vi "LoggingHeaders.vi"(7 "Match Number":u32, 8 "error in":errorcluster, 9 "Battery Number":string, 10 "Date and Time":string, 11 "refnum in":refnum<file>) -> (0 "error out":errorcluster, 3 "refnum out":refnum<file>)   [LabVIEW 2017]
uses:
  <vilib>/Rock Robotics/Network Tables/NT Read Number.vi
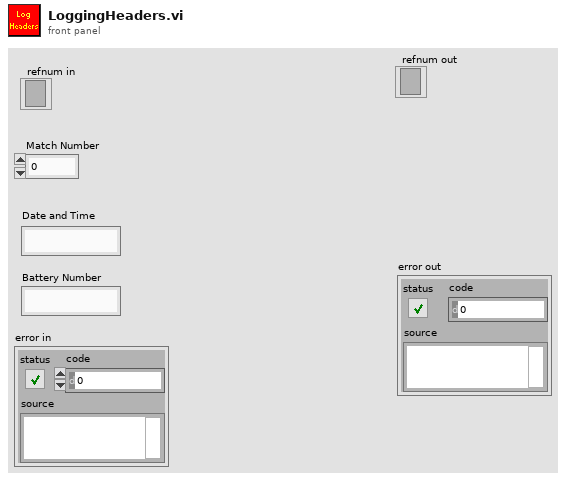
[diagram p1: front panel]
types:
  T1 = typedef "NetComm_MatchType.ctl" = enum32{"None", "Practice", "Qualification", "Elimination"}
  T2 = typedef "WPI_DriverStationPositionInfo.ctl" = enum16{"1", "2", "3"}
  T3 = typedef "WPI_DriverStationAllianceInfo.ctl" = enum16{"Red", "Blue", "Invalid"}
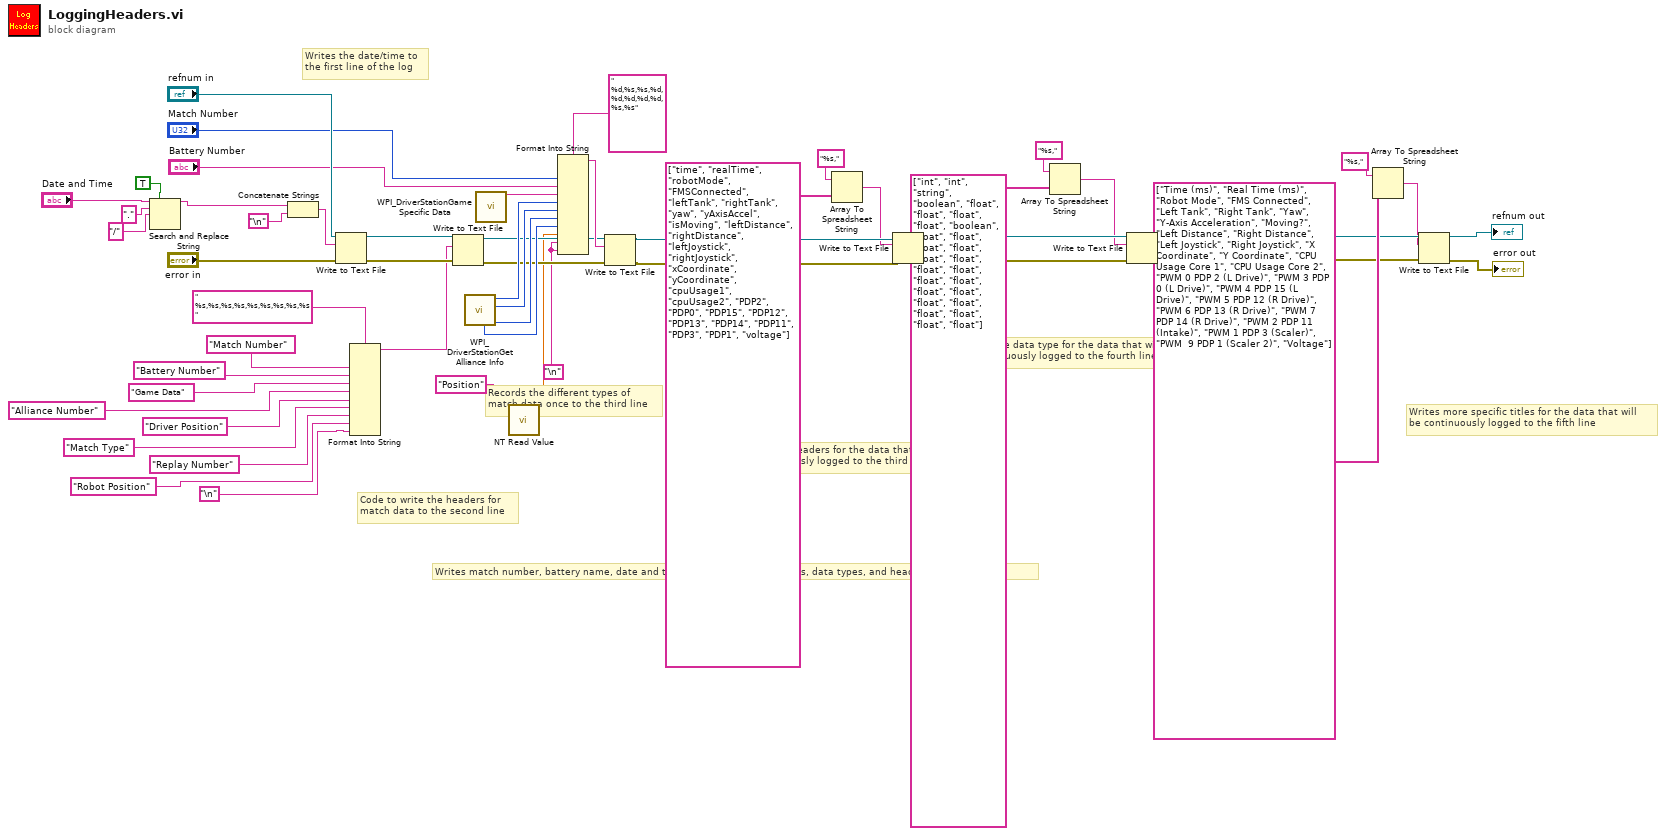
[diagram p0: block diagram]
diagram:
  w1 = "\n"
  # "Writes more specific titles for the data that will \nbe continuously logged to the fifth line"
  # "Writes the data type for the data that will \nbe continuously logged to the fourth line"
  # "Writes the headers for the data that will \nbe continuously logged to the third line"
  # "Records the different types of \nmatch data once to the third line"
  # "Code to write the headers for \nmatch data to the second line"
  # "Writes the date/time to\nthe first line of the log"
  # "Writes match number, battery name, date and time, headers variable names, data types, and headers to the log file"
  n1 = Search and Replace String(replace all?=TRUE ("replace all? (F)"), input string="Date and Time", search string=".", replace string="/" ("search string")) -> (result string=w6:string)  [unwired: 4 in, 3 out]
  n2 = Concatenate Strings(w6, "\n") -> (w52:string)
  n3 = Write to Text File(file (use dialog)="refnum in", text=w52, error in="error in") -> (refnum out=w23:refnum<file>, error out=w22:errorcluster)  [unwired: 1 in, 1 out]
  n4 = Format Into String(format string=" %s,%s,%s,%s,%s,%s,%s,%s,%s", "Match Number" ("input 2"), "Battery Number" ("input 2"), "Game Data" ("input 2"), "Alliance Number" ("input 2"), "Driver Position" ("input 2"), "Match Type" ("input 2"), "Replay Number" ("input 2"), "Robot Position" ("input 2"), "\n") -> (resulting string=w11:string)  [unwired: 2 in, 1 out]
  n5 = Write to Text File(file (use dialog)=w23, text=w11, error in=w22) -> (refnum out=w20:refnum<file>, error out=w21:errorcluster)  [unwired: 1 in, 1 out]
  n6 = call <vilib>:"WPI_DriverStationGet Alliance Info.vi"() -> ("Match Type"=w25:T1, "Position"=w26:T2, "Alliance"=w27:T3, "Replay Number"=w24:u16)  [unwired: 6 in, 2 out]
  n7 = call <vilib>:"WPI_DriverStationGame Specific Data.vi"() -> ("Game Specific Data"=w28:string)  [unwired: 11 in]
  n8 = call-poly <vilib>:"NT Read Value.vi"("Name"="Position") -> ("Numeric"=w2:dbl)  [unwired: 9 in, 1 out]
  n9 = Format Into String(format string=" %d,%s,%s,%d,%d,%d,%d,%d,%s,%s", "Match Number", "Battery Number", w28, w27, w26, w25, w24, w2, w1, w1) -> (resulting string=w48:string)  [unwired: 2 in, 1 out]
  n10 = Write to Text File(file (use dialog)=w20, text=w48, error in=w21) -> (refnum out=w41:refnum<file>, error out=w40:errorcluster)  [unwired: 1 in, 1 out]
  n11 = Array To Spreadsheet String(array=string[] ["time", "realTime", "robotMode", "FMSConnected", "leftTank", "rightTank", "yaw", "yAxisAccel", "isMoving", "leftDistance", "rightDistance", "leftJoystick", "rightJoystick", "xCoordinate", "yCoordinate", "cpuUsage1", "cpuUsage2", "PDP2", "PDP0", "PDP15", "PDP12", "PDP13", "PDP14", "PDP11", "PDP3", "PDP1", "voltage"], 3:"%s," ("format string")) -> (spreadsheet string=w33:string)  [unwired: 1 in]
  n12 = Write to Text File(file (use dialog)=w41, text=w33, error in=w40) -> (refnum out=w43:refnum<file>, error out=w42:errorcluster)  [unwired: 1 in, 1 out]
  n13 = Array To Spreadsheet String(array=string[] ["int", "int", "string", "boolean", "float", "float", "float", "float", "boolean", "float", "float", "float", "float", "float", "float", "float", "float", "float", "float", "float", "float", "float", "float", "float", "float", "float", "float"], 3:"%s," ("format string")) -> (spreadsheet string=w32:string)  [unwired: 1 in]
  n14 = Write to Text File(file (use dialog)=w43, text=w32, error in=w42) -> (refnum out=w37:refnum<file>, error out=w36:errorcluster)  [unwired: 1 in, 1 out]
  n15 = Array To Spreadsheet String(array=string[] ["Time (ms)", "Real Time (ms)", "Robot Mode", "FMS Connected", "Left Tank", "Right Tank", "Yaw", "Y-Axis Acceleration", "Moving?", "Left Distance", "Right Distance", "Left Joystick", "Right Joystick", "X Coordinate", "Y Coordinate", "CPU Usage Core 1", "CPU Usage Core 2", "PWM 0 PDP 2 (L Drive)", "PWM 3 PDP 0 (L Drive)", "PWM 4 PDP 15 (L Drive)", "PWM 5 PDP 12 (R Drive)", "PWM 6 PDP 13 (R Drive)", "PWM 7 PDP 14 (R Drive)", "PWM 2 PDP 11 (Intake)", "PWM 1 PDP 3 (Scaler)", "PWM  9 PDP 1 (Scaler 2)", "Voltage"], 3:"%s," ("format string")) -> (spreadsheet string=w31:string)  [unwired: 1 in]
  n16 = Write to Text File(file (use dialog)=w37, text=w31, error in=w36) -> (refnum out=→"refnum out":refnum<file>, error out=→"error out":errorcluster)  [unwired: 1 in, 1 out]
